vi "ChangeLanguage_test.vi"(10 "LanguageSelection":u16(ring) items=["Dansk", "English", "French"]) -> ()   [LabVIEW 2013, in "main.lvlib"]
uses:
  main.lvlib
  <vilib>/Utility/file.llb/Read From Spreadsheet File (string).vi
panel:
  out "appended array 2":string[](array[string])
  out "Array 2":string[](array[string])
  out "appended array":string[][](array[string])
  out "Array":string[][](array[string])
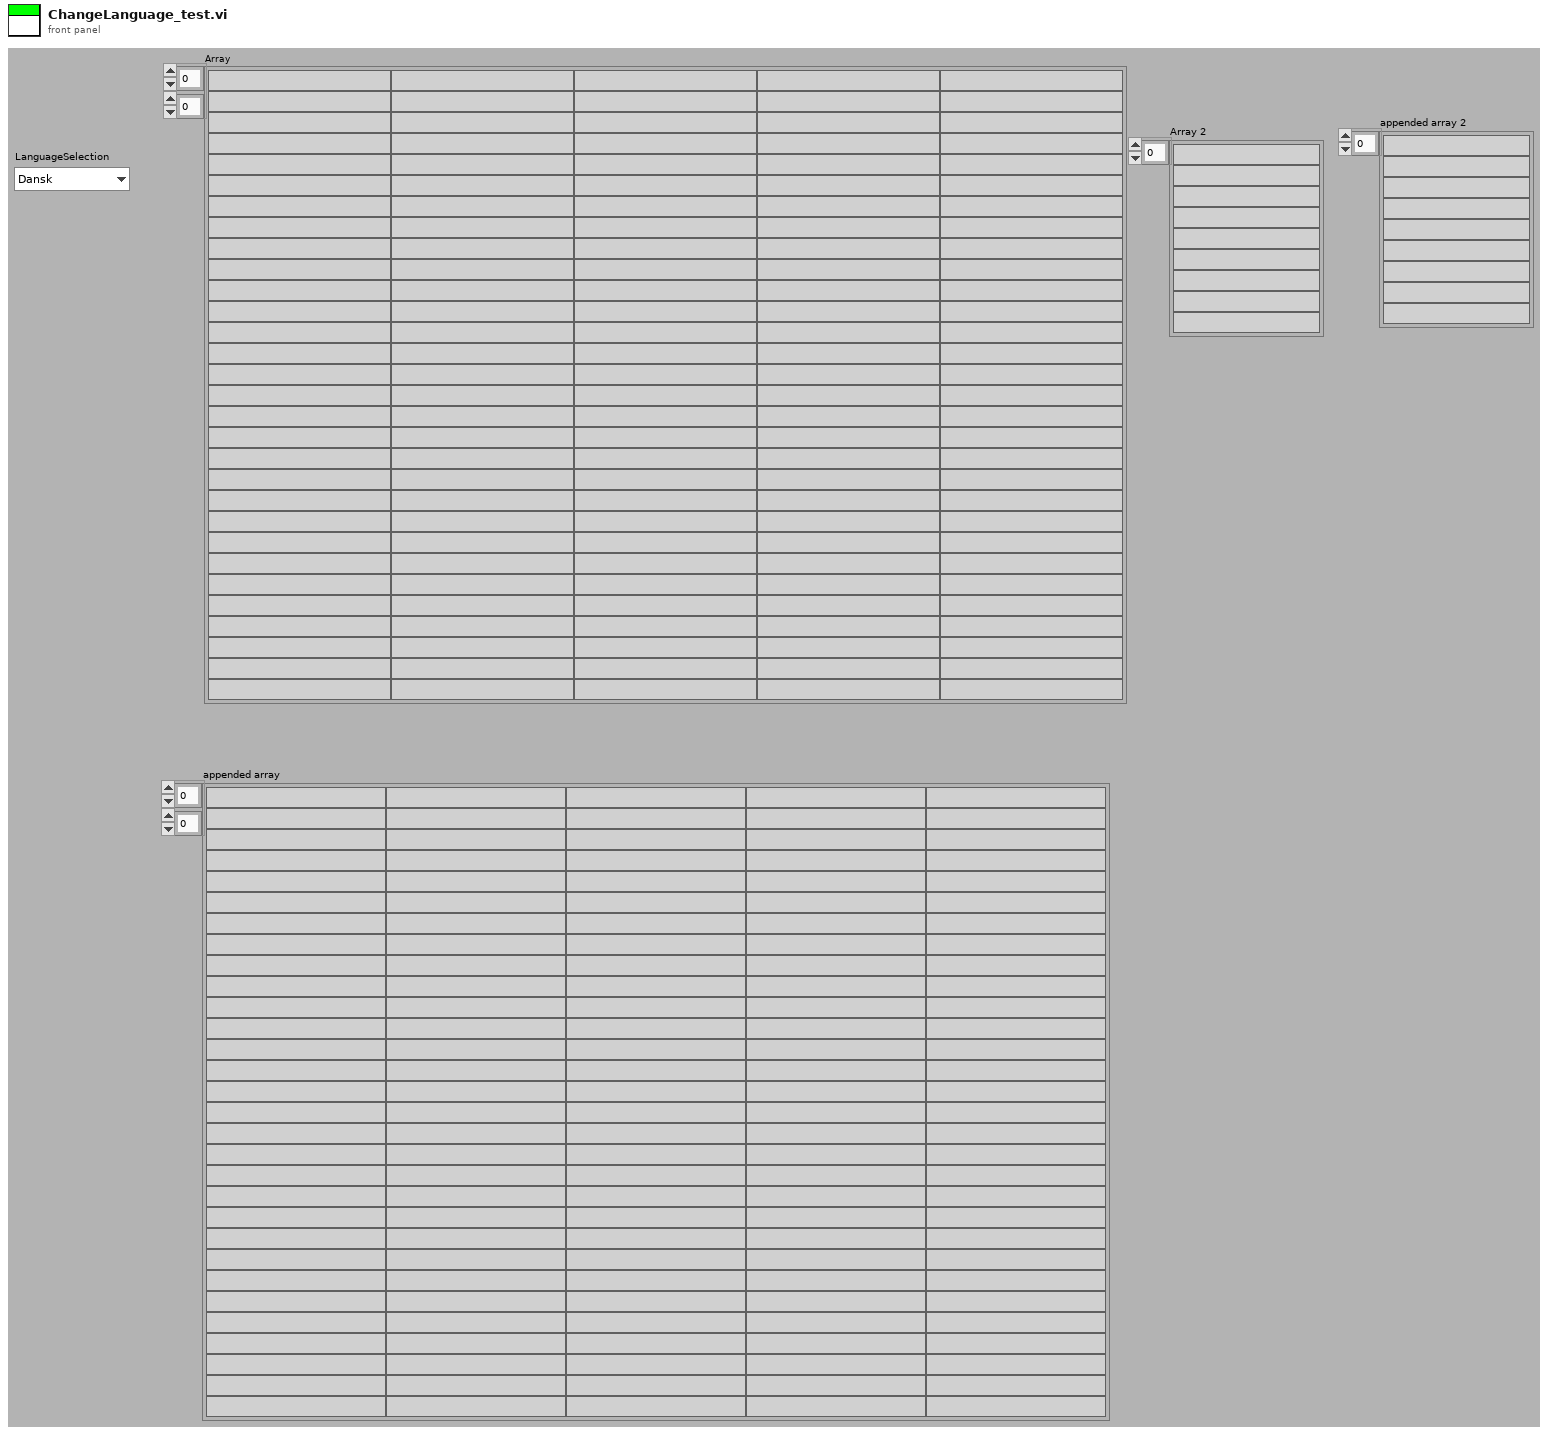
[diagram p1: front panel]
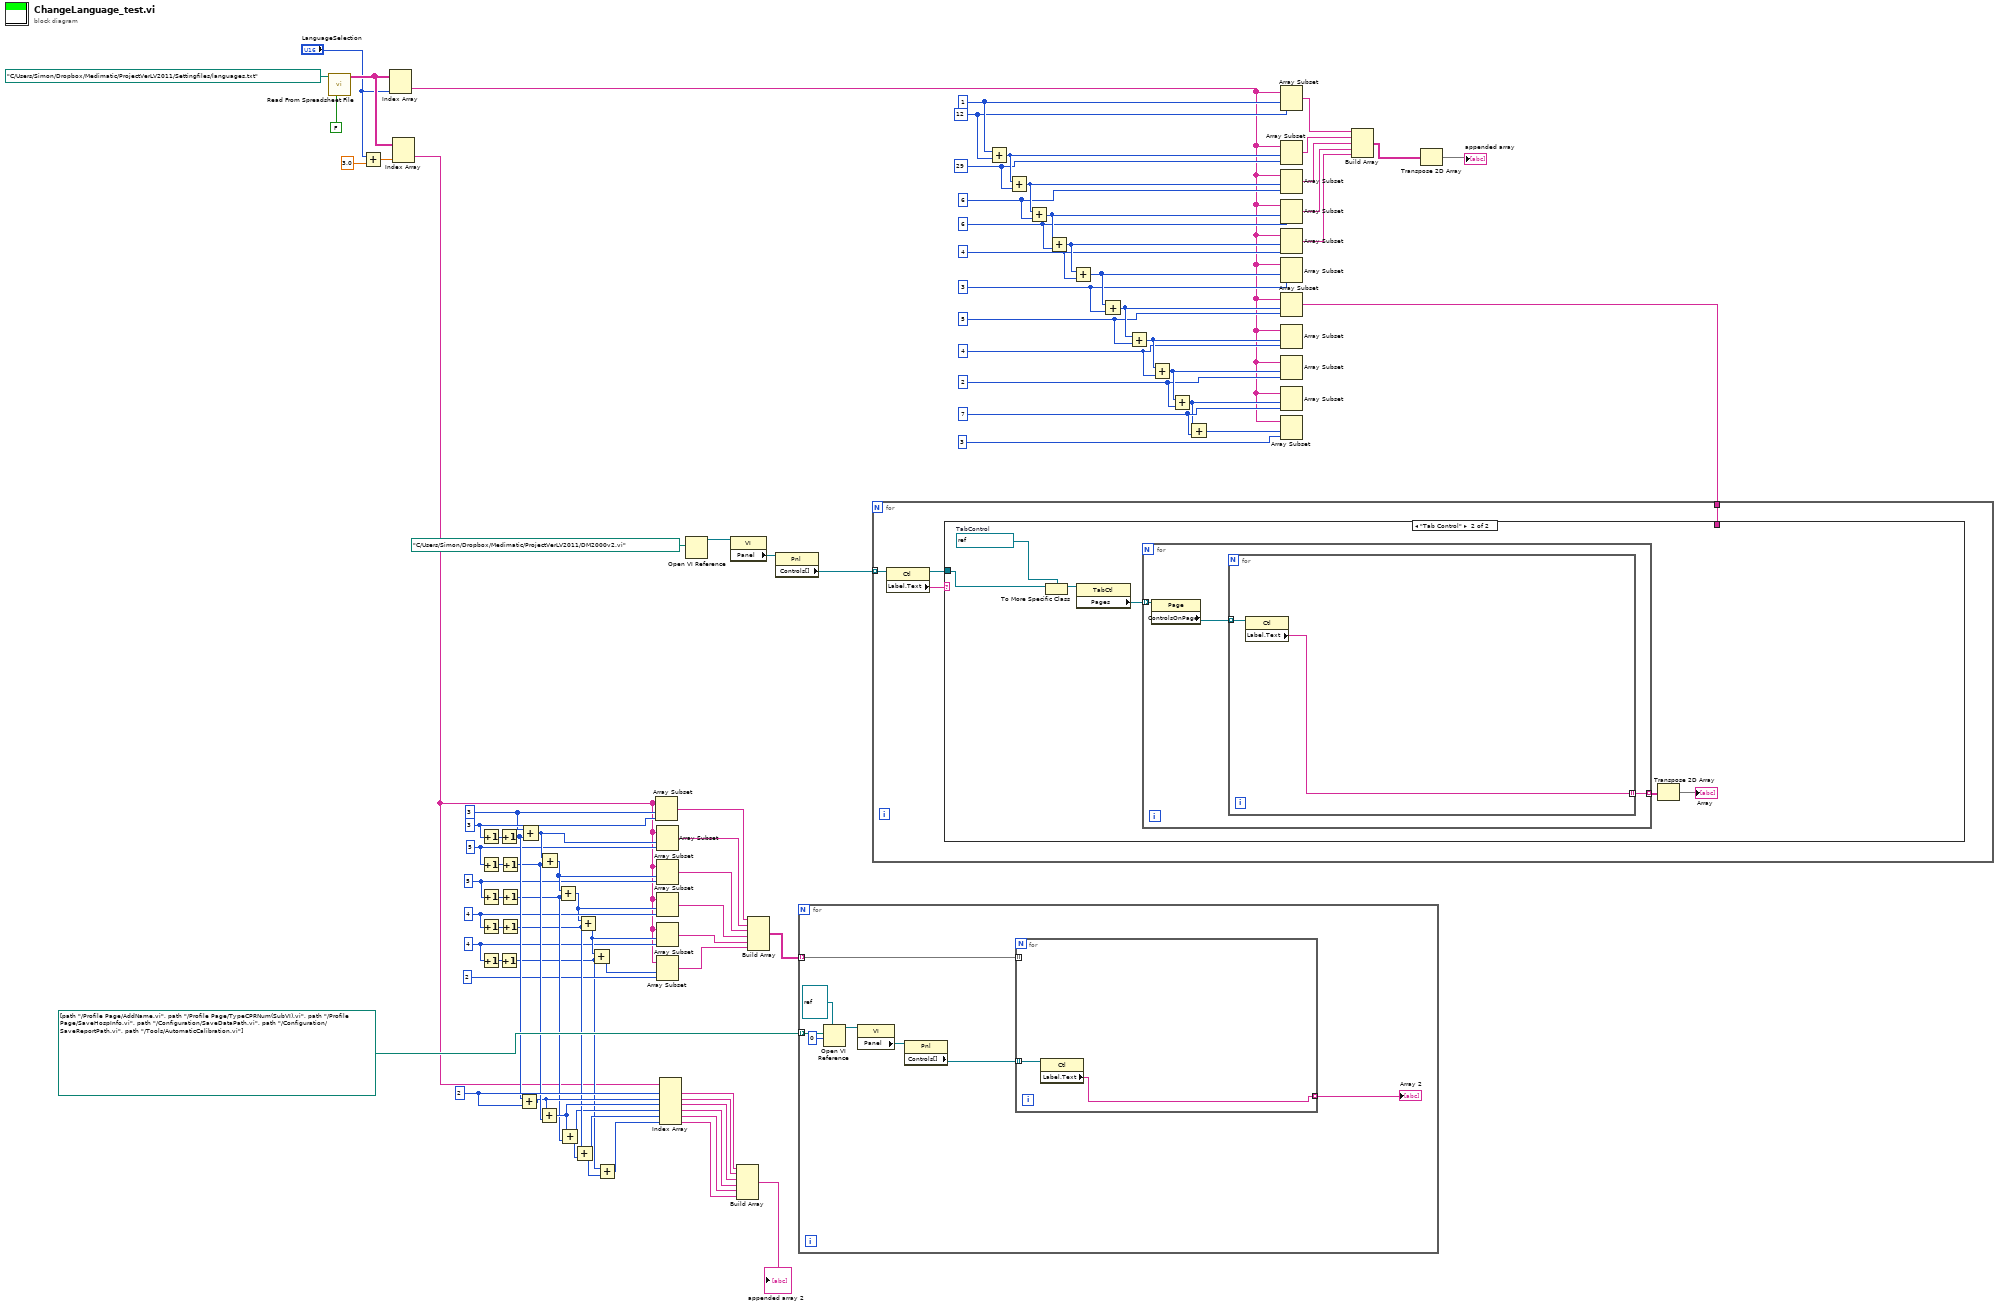
[diagram p0: block diagram]
diagram:
  w7 = 7
  w10 = 2
  w12 = 4
  w21 = 4 ("length")
  w32 = 4 ("length")
  w38 = 5 ("length")
  w45 = 5 ("length")
  w51 = 2 ("index")
  w50 = 3 ("length")
  w49 = 3 ("index")
  w14 = 5 ("length")
  w70 = 6 ("length")
  w72 = 29
  w64 = 3 ("length")
  w66 = 4 ("length")
  w68 = 6 ("length")
  w74 = 12 ("length")
  w75 = 1 ("index")
  n1 = call-poly <vilib>:"Read From Spreadsheet File.vi"("transpose (no:F)"=FALSE, "file path (dialog if empty)"=path "C:/Users/Simon/Dropbox/Medimatic/ProjectVerLV2011/Settingfiles/languages.txt") -> ("all rows"=w62:string[][])  [unwired: 5 in, 4 out]
  n2 = Add(x="LanguageSelection", y=3.0) -> (x+y=w61:dbl)
  n3 = Index Array(array=w62, index (col)="LanguageSelection") -> (element=w5:string[])  [unwired: 1 in]
  n4 = Index Array(array=w62, index (col)=w61) -> (element=w16:string[])  [unwired: 1 in]
  n5 = Increment(x=w50) -> (x+1=w52:i32)
  n6 = Increment(x=w21) -> (x+1=w25:i32)
  n7 = Increment(x=w45) -> (x+1=w47:i32)
  n8 = Increment(x=w38) -> (x+1=w40:i32)
  n9 = Increment(x=w32) -> (x+1=w33:i32)
  n10 = Increment(x=w52) -> (x+1=w48:i32)
  n11 = Increment(x=w25) -> (x+1=w20:i32)
  n12 = Increment(x=w47) -> (x+1=w43:i32)
  n13 = Increment(x=w40) -> (x+1=w36:i32)
  n14 = Increment(x=w33) -> (x+1=w30:i32)
  n15 = Add(x=w48, y=w51) -> (x+y=w42:i32)
  n16 = Add(x=w49, y=w48) -> (x+y=w46:i32)
  n17 = Add(x=w42, y=w43) -> (x+y=w37:i32)
  n18 = Add(x=w46, y=w43) -> (x+y=w39:i32)
  n19 = Add(x=w39, y=w36) -> (x+y=w31:i32)
  n20 = Add(x=w37, y=w36) -> (x+y=w29:i32)
  n21 = Add(x=w30, y=w29) -> (x+y=w26:i32)
  n22 = Add(x=w31, y=w30) -> (x+y=w22:i32)
  n23 = Add(x=w22, y=w20) -> (x+y=w23:i32)
  n24 = Add(x=w20, y=w26) -> (x+y=w19:i32)
  n25 = Array Subset(array=w16, index=w49, length=w50) -> (w58:string[])
  n26 = Array Subset(array=w16, index=w46, length=w45) -> (w57:string[])
  n27 = Array Subset(array=w16, index=w23, length=2) -> (w17:string[])
  n28 = Array Subset(array=w16, index=w39, length=w38) -> (w44:string[])
  n29 = Array Subset(array=w16, index=w31, length=w32) -> (w34:string[])
  n30 = Array Subset(array=w16, index=w22, length=w21) -> (w27:string[])
  n31 = Index Array(array=w16, index #1=w51, index #2=w42, index #3=w37, index #4=w29, index #5=w26, index #6=w19) -> (element #1=w54:string, element #2=w53:string, element #3=w41:string, element #4=w35:string, element #5=w28:string, element #6=w18:string)
  n32 = Open VI Reference(vi path=path "C:/Users/Simon/Dropbox/Medimatic/ProjectVerLV2011/DM2000v2.vi") -> (vi reference=w2:refnum<vi>)  [unwired: 5 in, 1 out]
  n33 = property class="VI"(reference=w2) -> ("Panel"=w85:refnum<vi>)  [unwired: 1 in, 2 out]
  n34 = Build Array(w54, w53, w41, w35, w28, w18) -> (→"appended array 2":string[])
  n35 = Build Array(w58, w57, w44, w34, w27, w17) -> (w55:string[][])
  n36 = property class="Pnl"(reference=w85) -> ("Controls[]"=w84:refnum<vi>[])  [unwired: 1 in, 2 out]
  n37 = for {
    tunnel: path[] [path "../Profile Page/AddName.vi", path "../Profile Page/TypeCPRNum(SubVI).vi", path "../Profile Page/SaveHospInfo.vi", path "../Configuration/SaveDataPath.vi", path "../Configuration/SaveReportPath.vi", path "../Tools/AutomaticCalibration.vi"] -> [w93] mode=indexing
    tunnel: w55 -> [w86] mode=indexing
    n38 = Open VI Reference(type specifier VI Refnum (for type only)=refnum<vi> refnum, vi path=w93, options=0) -> (vi reference=w87:refnum<vi>)  [unwired: 3 in, 1 out]
    n39 = property class="VI"(reference=w87) -> ("Panel"=w90:refnum<vi>)  [unwired: 1 in, 2 out]
    n40 = property class="Pnl"(reference=w90) -> ("Controls[]"=w92:refnum<vi>[])  [unwired: 1 in, 2 out]
    n41 = for {
      tunnel: w92 -> [w95] mode=indexing
      tunnel: [w94] -> w91 mode=indexing
      tunnel: w86 -> [_] mode=indexing
      n42 = property class="Ctl"(reference=w95) -> ("Label.Text"=w94:string)  [unwired: 1 in, 2 out]
    }
    "Array 2" <- w91
  }
  n43 = Add(x=w75, y=w74) -> (x+y=w73:i32)
  n44 = Add(x=w73, y=w72) -> (x+y=w71:i32)
  n45 = Add(x=w71, y=w70) -> (x+y=w69:i32)
  n46 = Add(x=w69, y=w68) -> (x+y=w67:i32)
  n47 = Add(x=w67, y=w66) -> (x+y=w65:i32)
  n48 = Add(x=w65, y=w64) -> (x+y=w15:i32)
  n49 = Add(x=w15, y=w14) -> (x+y=w13:i32)
  n50 = Add(x=w13, y=w12) -> (x+y=w11:i32)
  n51 = Add(x=w11, y=w10) -> (x+y=w6:i32)
  n52 = Add(x=w6, y=w7) -> (x+y=w9:i32)
  n53 = Array Subset(array=w5, index=w9, length=3) -> ()  [unwired: 1 out]
  n54 = Array Subset(array=w5, index=w75, length=w74) -> (w82:string[])
  n55 = Array Subset(array=w5, index=w73, length=w72) -> (w81:string[])
  n56 = Array Subset(array=w5, index=w71, length=w70) -> (w80:string[])
  n57 = Array Subset(array=w5, index=w69, length=w68) -> (w79:string[])
  n58 = Array Subset(array=w5, index=w67, length=w66) -> (w78:string[])
  n59 = Array Subset(array=w5, index=w65, length=w64) -> ()  [unwired: 1 out]
  n60 = Array Subset(array=w5, index=w15, length=w14) -> (w63:string[])
  n61 = for {
    tunnel: w84 -> [w99] mode=indexing
    tunnel: w63 -> [w96]
    n62 = property class="Ctl"(reference=w99) -> (reference out=w98:refnum<vi>, "Label.Text"=w97:string)  [unwired: 1 in, 1 out]
    n63 = case shown="\"Tab Control\"" w97 {
      tunnel: w98 -> [_ w105]
      tunnel: w96 -> [_ _]
      frame "False", Default {
      }
      frame "Tab Control" {
        w104 = refnum<vi> refnum  # TabControl
        n64 = To More Specific Class(target class=w104, reference=w105) -> (specific class reference=w103:refnum<vi>)  [unwired: 1 in, 1 out]
        n65 = property class="TabCtl"(reference=w103) -> ("Pages"=w100:refnum<vi>[])  [unwired: 1 in, 2 out]
        n66 = for {
          tunnel: w100 -> [w106] mode=indexing
          tunnel: [w107] -> w102 mode=indexing
          n67 = property class="Page"(reference=w106) -> ("ControlsOnPage"=w108:refnum<vi>[])  [unwired: 1 in, 2 out]
          n68 = for {
            tunnel: w108 -> [w110] mode=indexing
            tunnel: [w109] -> w107 mode=indexing
            n69 = property class="Ctl"(reference=w110) -> ("Label.Text"=w109:string)  [unwired: 1 in, 2 out]
          }
        }
        n70 = Transpose 2D Array(2D array=w102) -> (transposed array=→"Array":string[][])
      }
    }
  }
  n71 = Array Subset(array=w5, index=w13, length=w12) -> ()  [unwired: 1 out]
  n72 = Array Subset(array=w5, index=w11, length=w10) -> ()  [unwired: 1 out]
  n73 = Array Subset(array=w5, index=w6, length=w7) -> ()  [unwired: 1 out]
  n74 = Build Array(w82, w81, w80, w79, w78) -> (w76:string[][])
  n75 = Transpose 2D Array(2D array=w76) -> (transposed array=→"appended array":string[][])
